vi "Init Wind.vi"() -> (3 "Wind Queue Cluster":T1)   [LabVIEW 2013]
uses:
  Data/TypeDefs/WindData Queue Cluster.ctl
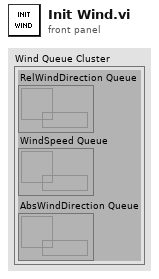
[diagram p1: front panel]
types:
  T1 = typedef "WindData Queue Cluster.ctl" = cluster{"RelWindDirection Queue":refnum<queue>, "WindSpeed Queue":refnum<queue>, "AbsWindDirection Queue":refnum<queue>}
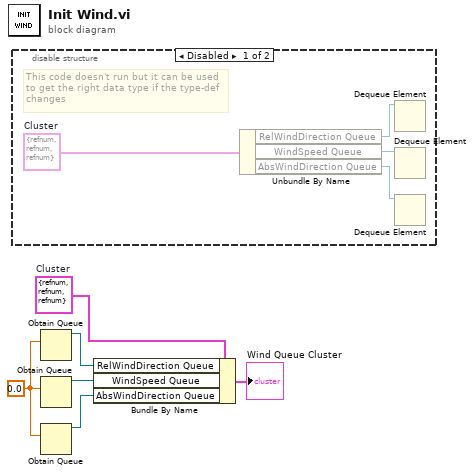
[diagram p0: block diagram]
diagram:
  w2 = 0.0 ("x")
  w6 = T1 {"RelWindDirection Queue"=refnum, "WindSpeed Queue"=refnum, "AbsWindDirection Queue"=refnum}  # Cluster
  n1 = disable-structure shown="Disabled" {
    frame Disabled {
      w8 = T1 {"RelWindDirection Queue"=refnum, "WindSpeed Queue"=refnum, "AbsWindDirection Queue"=refnum}  # Cluster
      # "This code doesn't run but it can be used to get the right data type if the type-def changes"
      n2 = Unbundle By Name(w8) -> ("RelWindDirection Queue"=w10:refnum<queue>, "WindSpeed Queue"=w9:refnum<queue>, "AbsWindDirection Queue"=w7:refnum<queue>)
      n3 = Dequeue Element(queue=w10) -> ()  [unwired: 2 in, 4 out]
      n4 = Dequeue Element(queue=w9) -> ()  [unwired: 2 in, 4 out]
      n5 = Dequeue Element(queue=w7) -> ()  [unwired: 2 in, 4 out]
    }
    frame Enabled {
    }
  }
  n6 = Obtain Queue ("AirmarGPS-Compass Queue")(element data type=w2) -> (queue out=w5:refnum<queue>)  [unwired: 4 in, 2 out]
  n7 = Obtain Queue ("AirmarGPS-Compass Queue")(element data type=w2) -> (queue out=w4:refnum<queue>)  [unwired: 4 in, 2 out]
  n8 = Obtain Queue ("AirmarGPS-Compass Queue")(element data type=w2) -> (queue out=w1:refnum<queue>)  [unwired: 4 in, 2 out]
  n9 = Bundle By Name(cluster=w6, "RelWindDirection Queue"=w5, "WindSpeed Queue"=w4, "AbsWindDirection Queue"=w1) -> (→"Wind Queue Cluster":T1)
